vi "Load DAC Configuration.vi"(8 "error in":errorcluster, 10 "Config File refnum in":T1, 11 "DAC TC Temperature in":refnum<class "DAC TC Temp CryoSep.lvclass">) -> (0 "error out":errorcluster, 2 "Config File refnum out":T1, 3 "DAC TC Temperature out":refnum<class "DAC TC Temp CryoSep.lvclass">)   [LabVIEW 2019, in "DAC.lvlib" / "DAC TC Temp CryoSep.lvclass"]
uses:
  DAC TC Temp CryoSep.lvclass
  C:/Users/krio/Documents/LV_Projects/test-stand/App/DAC/DAC.lvclass
  <vilib>/Utility/config.llb/Config Data RefNum.ctl
  DAC.lvclass/DAC.ctl
  DAC TC Temp CryoSep.lvclass/DAC TC Temp CryoSep.ctl
  <vilib>/Utility/config.llb/Read Key (String).vi
  DAC.lvclass
  <vilib>/Utility/config.llb/NI_LVConfig.lvlib
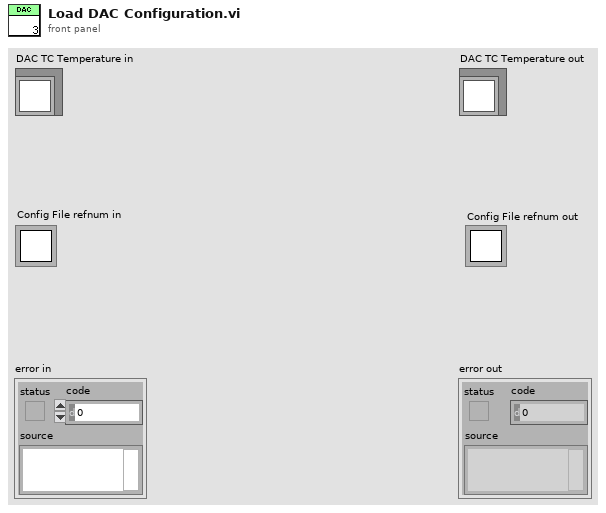
[diagram p1: front panel]
types:
  T1 = typedef "NI_LVConfig.lvlib/Config Data RefNum.ctl" = refnum<k1>
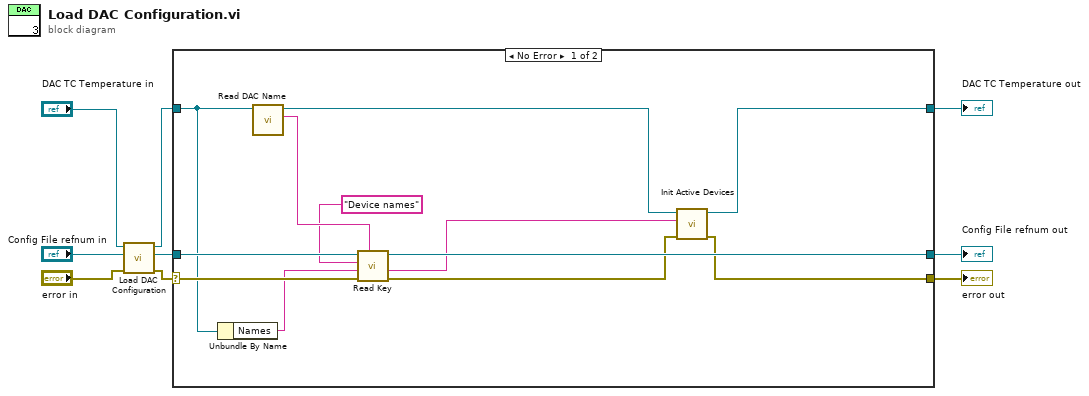
[diagram p0: block diagram]
diagram:
  n1 = call-parent "Load DAC Configuration.vi"("error in"="error in", "Config File refnum in"="Config File refnum in", "DAC in"="DAC TC Temperature in") -> ("error out"=w4:errorcluster, "Config File refnum out"=w5:T1, "DAC out"=w6:refnum<class "DAC TC Temp CryoSep.lvclass">)  [unwired: 6 in]
  n2 = case shown="No Error" w4 {
    selector: w4 -> [w19 w24]
    tunnel: [w10 w24] -> w1
    tunnel: [w13 w23] -> w3
    tunnel: w6 -> [w16 w23]
    tunnel: w5 -> [w21 w22]
    tunnel: [w20 w22] -> w2
    frame No Error {
      n3 = Unbundle By Name(w16) -> ("Names"=w15:string)
      n4 = call "Read DAC Name.vi"("DAC in"=w16) -> ("DAC Name"=w18:string, "DAC out"=w14:refnum<class "DAC TC Temp CryoSep.lvclass">)  [unwired: 8 in, 1 out]
      n5 = call-poly <vilib>:"Read Key.vi"("section"=w18, "error in (no error)"=w19, "default value"=w15, "key"="Device names", "refnum"=w21) -> ("error out"=w11:errorcluster, "value"=w12:string, "refnum out"=w20:T1)  [unwired: 3 in, 1 out]
      n6 = call "Init Active Devices.vi"("error in"=w11, "Device Names"=w12, "DAC TC Temperature in"=w14) -> ("error out"=w10:errorcluster, "DAC TC Temperature out"=w13:refnum<class "DAC TC Temp CryoSep.lvclass">)  [unwired: 7 in]
    }
    frame Error {
    }
  }
  "error out" <- w1
  "DAC TC Temperature out" <- w3
  "Config File refnum out" <- w2
